vi "Report Invalid Command.vi"(8 "Error In":errorcluster, 10 "Command":string, 11 "Process In":refnum<class "Process.lvclass">) -> (0 "Error Out":errorcluster, 3 "Process Out":refnum<class "Process.lvclass">)   [LabVIEW 2021, in "Process.lvclass"]
uses:
  Process.lvclass
  Central Message Handler/Public/Controls/Message.ctl
  <vilib>/Utility/error.llb/Error Cluster From Error Code.vi
  Accessors/Central Message Handler Queue/Get Central Message Handler Queue.vi
  <vilib>/ErrorRing/Error Ring.xnode
  Central Message Handler/Central Message Handler.lvclass
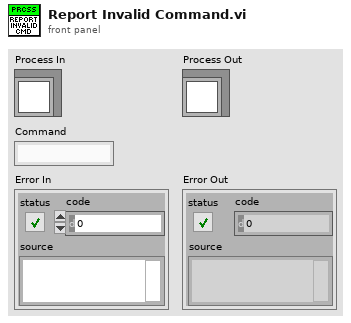
[diagram p1: front panel]
types:
  T1 = typedef "Central Message Handler.lvclass/Message.ctl" = cluster{"Command":string, "Data":variant, "Receiver":string}
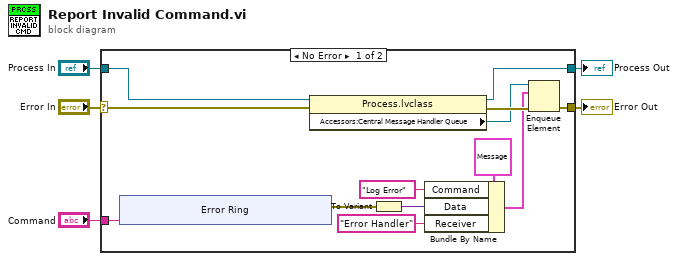
[diagram p0: block diagram]
diagram:
  n1 = case shown="No Error" "Error In" {
    selector: "Error In" -> [w8 w26]
    tunnel: [w9 w26] -> w4
    tunnel: "Process In" -> [w18 w27]
    tunnel: [w10 w27] -> w2
    tunnel: "Command" -> [w7 _]
    frame No Error {
      n2 = xnode "Error Ring"("parameter 0"=w7) -> ("error out"=w6:errorcluster)
      n3 = property class="Process.lvclass"(reference=w18, error in=w8) -> (reference out=w10:refnum<class "Process.lvclass">, error out=w17:errorcluster, "Accessors:Central Message Handler Queue"=w16:refnum<queue>)
      n4 = To Variant(anything=w6) -> (Variant=w14:variant)
      n5 = Bundle By Name(cluster=T1 {"Command"="", "Data"=variant, "Receiver"=""} ("element"), "Command"="Log Error", "Data"=w14, "Receiver"="Error Handler") -> (w11:T1)
      n6 = Enqueue Element(queue=w16, element=w11, error in (no error)=w17) -> (error out=w9:errorcluster)  [unwired: 1 in, 2 out]
    }
    frame Error {
    }
  }
  "Process Out" <- w2
  "Error Out" <- w4
